vi "GetText.vi"(8 "error in":errorcluster, 11 "node in":refnum<class "NISE_CEF_serializable node.lvclass">) -> (0 "error out":errorcluster, 1 "additional text":string, 2 "text":string, 3 "node out":refnum<class "NISE_CEF_serializable node.lvclass">, 4 "glyph":string)   [LabVIEW 2013, in "NISE_CEF_serializable node.lvclass"]
doc: "Returns the text representation of the node used for the tree control."
uses:
  NISE_CEF_serializable node.lvclass
  Node/NISE_CEF_Node.lvclass
  serializable configuration/NISE_CEF_serializable configuration.lvclass
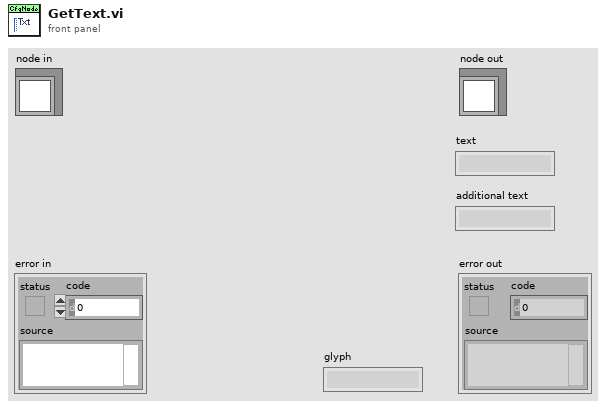
[diagram p1: front panel]
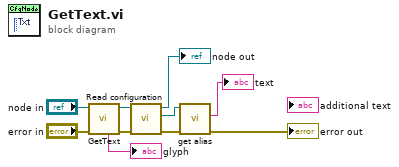
[diagram p0: block diagram]
diagram:
  n1 = call-parent "GetText.vi"("error in"="error in", "node in"="node in") -> ("error out"=w7:errorcluster, "node out"=w6:refnum<class "NISE_CEF_serializable node.lvclass">, "glyph"=→"glyph":string)  [unwired: 5 in, 2 out]
  n2 = call-dynamic "Read configuration.vi"("error in"=w7, "NISE_CEF_serializable node in"=w6) -> ("error out"=w4:errorcluster, "configuration"=w3:refnum<class "NISE_CEF_serializable configuration.lvclass">, "NISE_CEF_serializable node out"=→"node out":refnum<class "NISE_CEF_serializable node.lvclass">)  [unwired: 7 in]
  n3 = call "get alias.vi"("error in"=w4, "configuration in"=w3) -> ("error out"=→"error out":errorcluster, "alias"=→"text":string)  [unwired: 7 in, 1 out]
